vi "S.K.Y Controller.vi"   [LabVIEW 2019]
uses:
  <vilib>/Rock Robotics/WPI/Joystick/WPI_JoystickDeviceEnum.ctl
  S.K.Y Controller Global.vi
types:
  T1 = typedef "WPI_JoystickDeviceEnum.ctl" = enum16{"USB 0", "USB 1", "USB 2", "USB 3", "USB 4", "USB 5"}
  T2 = typedef "WPI_JoystickDevRef.ctl" = cluster{"Device":T1}
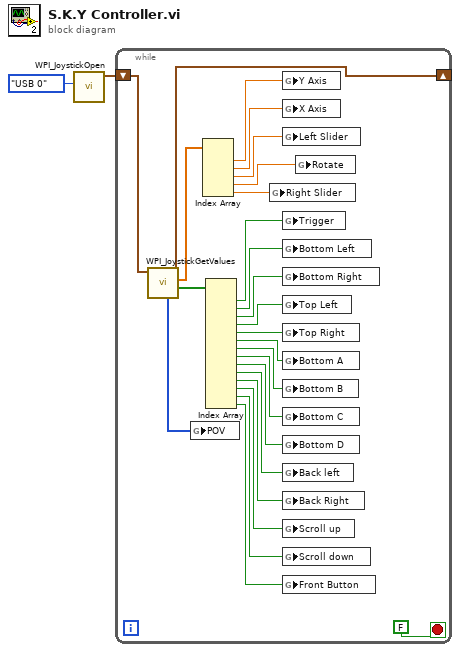
[diagram p0: block diagram]
diagram:
  n1 = call <vilib>:"WPI_JoystickOpen.vi"("JoystickDevice"=WPI_JoystickDeviceEnum."USB 0") -> ("JoystickDevRef"=w2:T2)  [unwired: 10 in]
  n2 = while {
    shift-right: [w25] -> _
    shift-left: w2 -> [w26]
    stop <- FALSE stop-if-true
    n3 = call <vilib>:"WPI_JoystickGetValues.vi"("JoystickDevRef"=w26) -> ("Buttons"=w24:bool[], "Axes"=w9:dbl[], "JoystickDevRef"=w25:T2, "POVs"=w3:i16[])  [unwired: 6 in, 1 out]
    n4 = global write "S.K.Y Controller Global.vi" "POV"(w3) -> ()
    n5 = Index Array(array=w9) -> (element #1=w8:dbl, element #2=w7:dbl, element #3=w6:dbl, element #4=w5:dbl, element #5=w4:dbl)  [unwired: 5 in]
    n6 = Index Array(array=w24) -> (element #1=w23:bool, element #2=w22:bool, element #3=w21:bool, element #4=w20:bool, element #5=w19:bool, element #6=w18:bool, element #7=w17:bool, element #8=w16:bool, element #9=w15:bool, element #10=w14:bool, element #11=w13:bool, element #12=w12:bool, element #13=w10:bool, element #14=w11:bool)  [unwired: 14 in]
    n7 = global write "S.K.Y Controller Global.vi" "Right Slider"(w4) -> ()
    n8 = global write "S.K.Y Controller Global.vi" "Y Axis"(w8) -> ()
    n9 = global write "S.K.Y Controller Global.vi" "X Axis"(w7) -> ()
    n10 = global write "S.K.Y Controller Global.vi" "Left Slider"(w6) -> ()
    n11 = global write "S.K.Y Controller Global.vi" "Trigger"(w23) -> ()
    n12 = global write "S.K.Y Controller Global.vi" "Bottom Left"(w22) -> ()
    n13 = global write "S.K.Y Controller Global.vi" "Bottom Right"(w21) -> ()
    n14 = global write "S.K.Y Controller Global.vi" "Top Left"(w20) -> ()
    n15 = global write "S.K.Y Controller Global.vi" "Top Right"(w19) -> ()
    n16 = global write "S.K.Y Controller Global.vi" "Bottom A"(w18) -> ()
    n17 = global write "S.K.Y Controller Global.vi" "Bottom B"(w17) -> ()
    n18 = global write "S.K.Y Controller Global.vi" "Bottom C"(w16) -> ()
    n19 = global write "S.K.Y Controller Global.vi" "Bottom D"(w15) -> ()
    n20 = global write "S.K.Y Controller Global.vi" "Back left"(w14) -> ()
    n21 = global write "S.K.Y Controller Global.vi" "Back Right"(w13) -> ()
    n22 = global write "S.K.Y Controller Global.vi" "Scroll up"(w12) -> ()
    n23 = global write "S.K.Y Controller Global.vi" "Scroll down"(w10) -> ()
    n24 = global write "S.K.Y Controller Global.vi" "Front Button"(w11) -> ()
    n25 = global write "S.K.Y Controller Global.vi" "Rotate"(w5) -> ()
  }
